vi "Copy Webroot to Apache Root Directory.vi"() -> ()   [LabVIEW 2020]
panel:
  out "filenames":string[](array[string])
  out "return code":i32
  out "standard error":string
  out "standard output":string
  out "permissions":i16
  out "group":string
  out "owner":string
  in  "error in (no error)":errorcluster
  out "error out":errorcluster
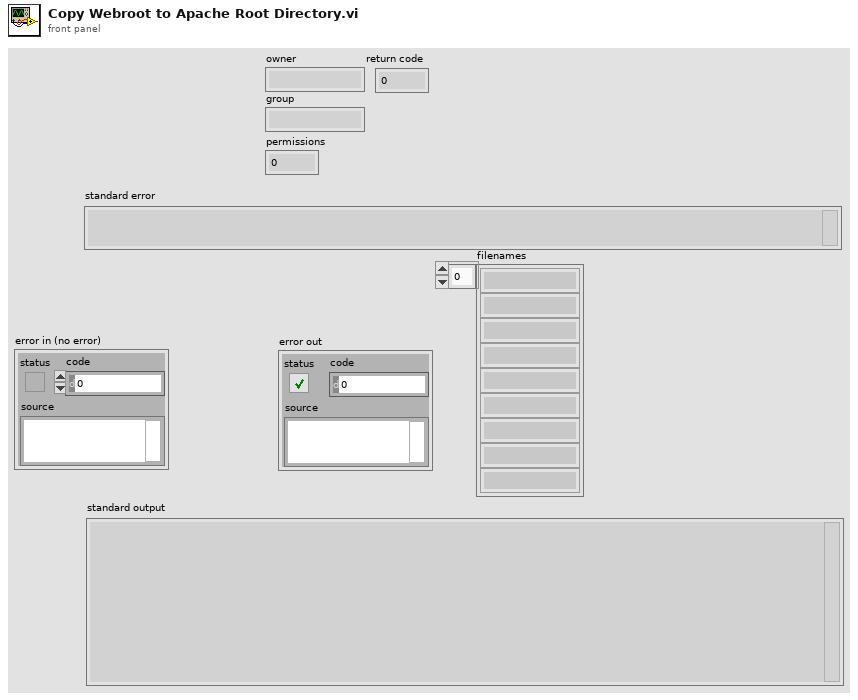
[diagram p1: front panel]
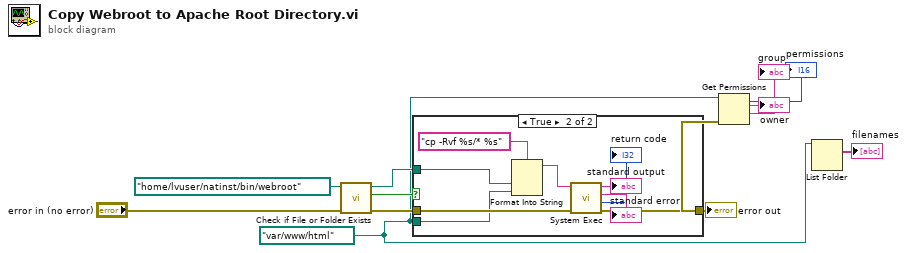
[diagram p0: block diagram]
diagram:
  w2 = path "/var/www/html" ("target path (use dialog)")
  n1 = call <vilib>:"Check if File or Folder Exists.vi"("error in (no error)"="error in (no error)", "path"=path "/home/lvuser/natinst/bin/webroot") -> ("error out"=w10:errorcluster, "file or folder exists?"=w9:bool, "dup path"=w7:path)  [unwired: 7 in]
  n2 = case shown="True" w9 {
    tunnel: w10 -> [w12 w20]
    tunnel: [w12 w21] -> w3
    tunnel: w7 -> [_ w19]
    tunnel: w2 -> [_ w18]
    frame False {
    }
    frame True {
      n3 = Format Into String(format string="cp -Rvf %s/* %s", w19, w18) -> (resulting string=w17:string)  [unwired: 2 in, 1 out]
      n4 = call <vilib>:"System Exec.vi"("error in (no error)"=w20, "command line"=w17) -> ("error out"=w21:errorcluster, "return code"=→"return code":i32, "standard error"=→"standard error":string, "standard output"=→"standard output":string)  [unwired: 6 in]
    }
  }
  "error out" <- w3
  n5 = Get Permissions(8:w3, 11:w2) -> (1:→"group":string, 2:→"owner":string, 5:→"permissions":i16)  [unwired: 2 out]
  n6 = List Folder(path=w2) -> (filenames=→"filenames":string[])  [unwired: 3 in, 3 out]
